vi "Grow Blob.vi"(4 "Blob Step":i16=-1, 5 "First Blob Value":i16=255, 6 "Error":string, 8 "Output Image":T1={"Image ID"=0, "Channel ID"=-1}, 9 "Input Image":T1={"Image ID"=0, "Channel ID"=-1}) -> (0 "Error":string, 2 "Output Image":T1={"Image ID"=0, "Channel ID"=-1}, 3 "Input Image":T1={"Image ID"=0, "Channel ID"=-1})   [LabVIEW 2011, in "labvvis.lvlib"]
doc: "Grows blobs. Treats 0 as background and any non-zero value as a foreground object. Grow Blob only operates on grey images. It does not work on any of the other single-channel images. To use Grow Blob with these images, you will need to Copy them to grey images.\n\nThe background is always labelled 0. Object blob labelling by default starts from 255 and decreases by 1 for each new blob. You can change these values by setting \"First Blob Value\" and \"Blob Step\". By default, \"First Blob Value\" is 255 and \"Blob Step\" is \"-1\".\n\nNote that due to the nature of the algorithm, not all blob labels within the range used will have non-zero region. Thus, you cannot just look for the lowest non-zero value, and subtract that from 255 to get the number of blobs. You will have to count the number of distinct values that are non-zero."
uses:
  <userlib>/labvvis/labvvis.lvlib
  labvvis.framework
  <userlib>/labvvis/VVIS Image.ctl
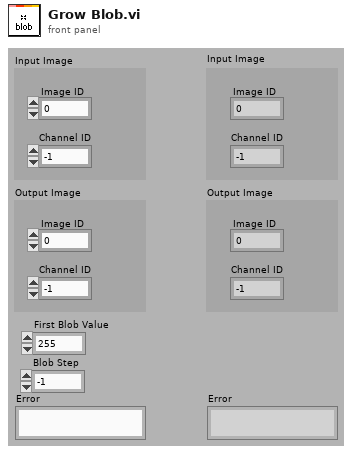
[diagram p1: front panel]
types:
  T1 = typedef "labvvis.lvlib/VVIS Image.ctl" = cluster{"Image ID":i16, "Channel ID":i16}
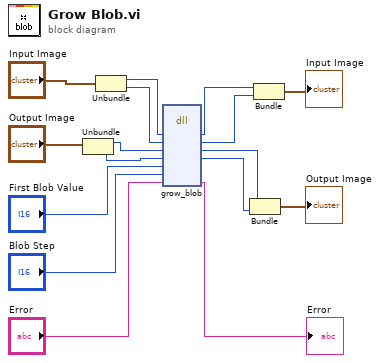
[diagram p0: block diagram]
diagram:
  n1 = Unbundle("Output Image") -> ("Image ID"=w12:i16, "Channel ID"=w11:i16)
  n2 = Unbundle("Input Image") -> ("Image ID"=w14:i16, "Channel ID"=w13:i16)
  n3 = dll-call lib="labvvis.framework" fn="grow_blob"("src1"=w14, "icid"=w13, "out"=w12, "ocid"=w11, "blob_start"="First Blob Value", "blob_step"="Blob Step", "Error") -> ("src1"=w3:i16, "icid"=w4:i16, "out"=w5:i16, "ocid"=w6:i16, →"Error":string)  [unwired: 6 in, 2 out]
  n4 = Bundle("out"=w5, "ocid"=w6) -> (→"Output Image":cluster{"out":i16, "ocid":i16})  [unwired: 1 in]
  n5 = Bundle("src1"=w3, "icid"=w4) -> (→"Input Image":cluster{"src1":i16, "icid":i16})  [unwired: 1 in]
